vi "GetChannelStatus.vi"(8 "error in (no error)":errorcluster, 11 "waveform in":waveform(sgl)) -> (0 "error out":errorcluster, 1 "t0":timestamp, 2 "channel status":string, 3 "waveform out":waveform(sgl))   [LabVIEW 2017, in "ChannelStatus.lvlib"]
uses:
  <vilib>/addons/InsightCM/Utilities/ChannelStatus/ChannelStatus.lvlib
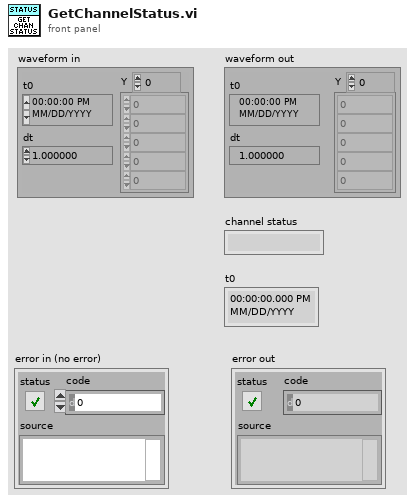
[diagram p1: front panel]
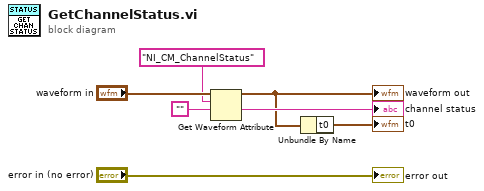
[diagram p0: block diagram]
diagram:
  n1 = Get Waveform Attribute(5:"", 6:"NI_CM_ChannelStatus" ("name"), 7:"waveform in") -> (1:→"channel status":string, 3:w4:waveform(sgl))  [unwired: 1 in, 2 out]
  "waveform out" <- w4
  n2 = Unbundle By Name(w4) -> ("t0"=→"t0":timestamp)
  "error out" <- "error in (no error)"
